vi "Get Video Mode.vi"(8 "error in (no error)":errorcluster, 11 "VISA resource name":refnum<visa-resource-name>) -> (0 "error out":errorcluster, 1 "Video Line Marker":i32, 2 "Video Format":i32, 3 "VISA resource name out":refnum<visa-resource-name>)   [LabVIEW 2014, in "Fluke 5XXX Series Multicalibrators.lvlib"]
doc: "This VI returns the format of Video scope mode and returns the Video mode line marker location.\n\nNote:\n\nThis VI is available only for instrument models 5500A and 5520A with oscilloscope option SC600 (SC1100)."
uses:
  Fluke 5XXX Series Multicalibrators.lvlib
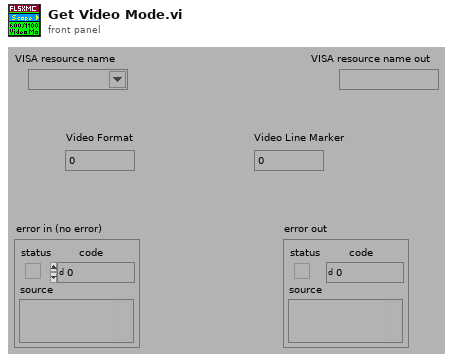
[diagram p1: front panel]
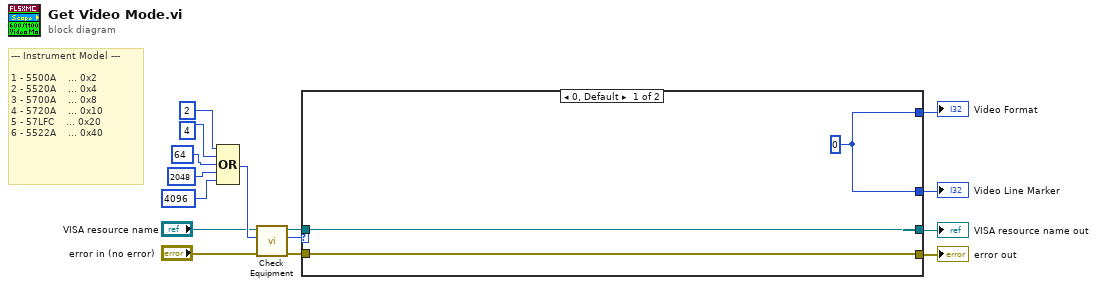
[diagram p0: block diagram]
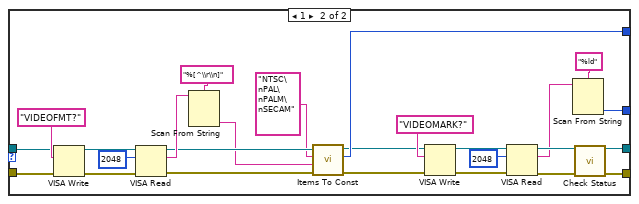
[diagram p2: hidden frame]
diagram:
  # "--- Instrument Model ---\n\n1 - 5500A    ... 0x2\n2 - 5520A    ... 0x4\n3 - 5700A    ... 0x8\n4 - 5720A    ... 0x10\n5 - 57LFC    ... 0x20\n6 - 5522A    ... 0x40"
  n1 = Compound Arithmetic op=OR(2 ("Numeric"), 4 ("Numeric"), 64 ("Numeric"), 2048 ("Numeric"), 4096 ("Numeric")) -> (w8:i32)
  n2 = call "Check Equipment.vi"("error in (no error)"="error in (no error)", "Bit Mask"=w8, "VISA resource name"="VISA resource name") -> ("error out"=w15:errorcluster, "Present?"=w14:u32, "VISA resource name out"=w13:refnum<visa-resource-name>)  [unwired: 6 in]
  n3 = case shown="0, Default" w14 {
    tunnel: [w18 w38] -> w5
    tunnel: [w17 w37] -> w4
    tunnel: w15 -> [w18 w40]
    tunnel: w13 -> [w17 w39]
    tunnel: [w16 w31] -> w2
    tunnel: [w16 w20] -> w3
    frame 0, Default {
      w16 = 0
    }
    frame 1 {
      n4 = VISA Write(VISA resource name=w39, write buffer="VIDEOFMT?", error in (no error)=w40) -> (VISA resource name out=w43:refnum<visa-resource-name>, error out=w42:errorcluster)  [unwired: 1 out]
      n5 = VISA Read(VISA resource name=w43, byte count=u32 2048 ("byte count (0)"), error in (no error)=w42) -> (VISA resource name out=w33:refnum<visa-resource-name>, read buffer=w35:string, error out=w34:errorcluster)  [unwired: 1 out]
      n6 = Scan From String(format string="%[^\\r\\n]", input string=w35) -> (output 1=w32:string)  [unwired: 3 in, 3 out]
      n7 = call "Items To Const.vi"("error in (no error)"=w34, "String Item"=w32, "Multi-Line String"="NTSC\nPAL\nPALM\nSECAM", "VISA resource name"=w33) -> ("error out"=w23:errorcluster, "Index"=w31:i32, "VISA resource name out"=w24:refnum<visa-resource-name>)  [unwired: 5 in]
      n8 = VISA Write(VISA resource name=w24, write buffer="VIDEOMARK?", error in (no error)=w23) -> (VISA resource name out=w29:refnum<visa-resource-name>, error out=w27:errorcluster)  [unwired: 1 out]
      n9 = VISA Read(VISA resource name=w29, byte count=u32 2048 ("byte count (0)"), error in (no error)=w27) -> (VISA resource name out=w25:refnum<visa-resource-name>, read buffer=w21:string, error out=w26:errorcluster)  [unwired: 1 out]
      n10 = Scan From String(format string="%ld", input string=w21) -> (output 1=w20:i32)  [unwired: 3 in, 3 out]
      n11 = call "Check Status.vi"("VISA resource name"=w25, "error in (no error)"=w26) -> ("VISA resource name out"=w37:refnum<visa-resource-name>, "error out"=w38:errorcluster)  [unwired: 12 in]
    }
  }
  "Video Format" <- w2
  "Video Line Marker" <- w3
  "VISA resource name out" <- w4
  "error out" <- w5
